vi "SetSplittersSticking.vi"(8 "error in (no error)":errorcluster, 9 "Horizontal Resizing":u16(ring)=1 items=["left", "middle", "right"], 10 "Vertical Resizing":u16(ring)=1 items=["top", "middle", "bottom"], 11 "Splitters":T1) -> (0 "error out":errorcluster)   [LabVIEW 2022 SP3, in "PentaPanesLibrary.lvlib" / "PentaPanes.lvclass"]
uses:
  PentaPanes.lvclass
  SplittersCluster.ctl
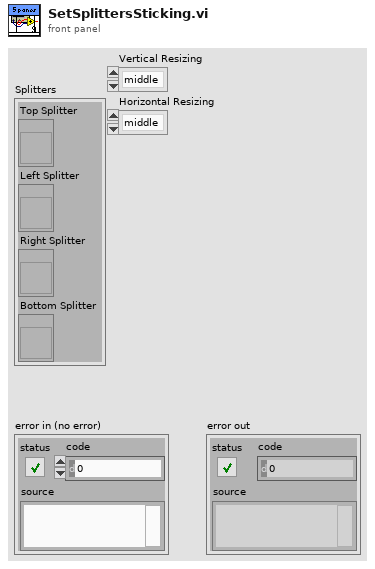
[diagram p1: front panel]
types:
  T1 = typedef "PentaPanesLibrary.lvlib/PentaPanes.lvclass/SplittersCluster.ctl" = cluster{"Top Splitter":refnum<vi>, "Left Splitter":refnum<vi>, "Right Splitter":refnum<vi>, "Bottom Splitter":refnum<vi>}
  T2 = enum16{"Sticks Top/Left", "Sticks Bottom/Right", "Proportional"}
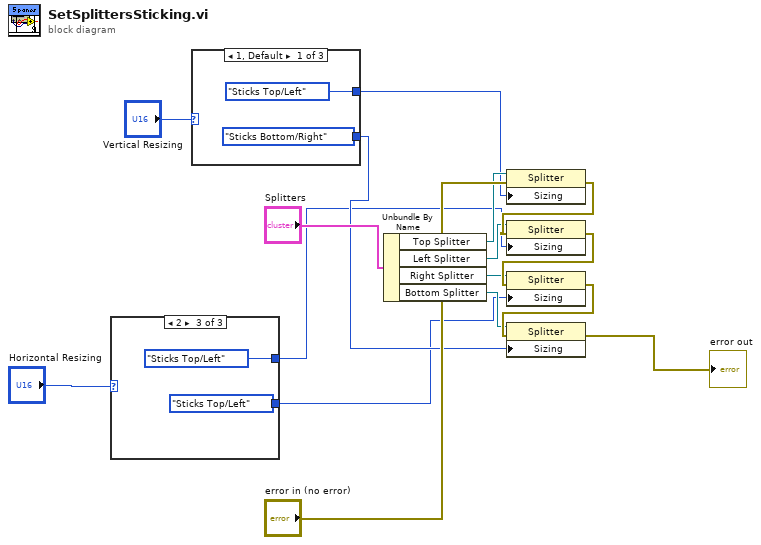
[diagram p0: block diagram]
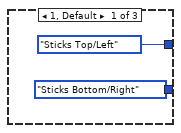
[diagram p2: hidden frame]
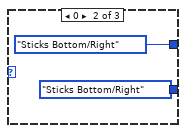
[diagram p3: hidden frame]
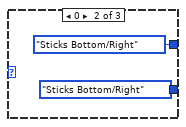
[diagram p4: hidden frame]
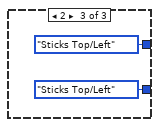
[diagram p5: hidden frame]
diagram:
  n1 = case shown="2" "Horizontal Resizing" {
    tunnel: [T2."Sticks Top/Left" ("Sizing") T2."Sticks Bottom/Right" ("Sizing") T2."Sticks Top/Left" ("Sizing")] -> w2
    tunnel: [T2."Sticks Bottom/Right" ("Sizing") T2."Sticks Bottom/Right" ("Sizing") T2."Sticks Top/Left" ("Sizing")] -> w1
    frame 1, Default {
    }
    frame 0 {
    }
    frame 2 {
    }
  }
  n2 = case shown="1, Default" "Vertical Resizing" {
    tunnel: [T2."Sticks Top/Left" ("Sizing") T2."Sticks Bottom/Right" ("Sizing") T2."Sticks Top/Left" ("Sizing")] -> w5
    tunnel: [T2."Sticks Bottom/Right" ("Sizing") T2."Sticks Bottom/Right" ("Sizing") T2."Sticks Top/Left" ("Sizing")] -> w4
    frame 1, Default {
    }
    frame 0 {
    }
    frame 2 {
    }
  }
  n3 = Unbundle By Name("Splitters") -> ("Top Splitter"=w7:refnum<vi>, "Left Splitter"=w8:refnum<vi>, "Right Splitter"=w9:refnum<vi>, "Bottom Splitter"=w10:refnum<vi>)
  n4 = property class="Splitter"(reference=w7, error in="error in (no error)", "Sizing"=w5) -> (error out=w11:errorcluster)  [unwired: 1 out]
  n5 = property class="Splitter"(reference=w8, error in=w11, "Sizing"=w2) -> (error out=w12:errorcluster)  [unwired: 1 out]
  n6 = property class="Splitter"(reference=w9, error in=w12, "Sizing"=w1) -> (error out=w13:errorcluster)  [unwired: 1 out]
  n7 = property class="Splitter"(reference=w10, error in=w13, "Sizing"=w4) -> (error out=→"error out":errorcluster)  [unwired: 1 out]
